vi "Echo Info.vi"(11 "Echo Info":string) -> (0 "Info Data":u16, 1 "Info Code":u16, 2 "FC":u8, 3 "Amplifier Num":u8, 4 "Check Result":bool)   [LabVIEW 2014, in "ALPHA5 RS485.lvlib"]
uses:
  ALPHA5 RS485.lvlib
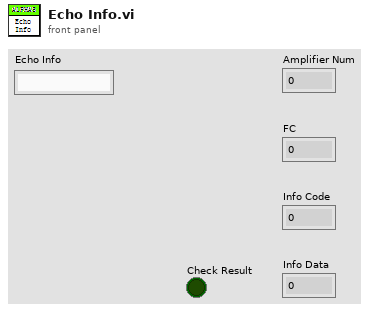
[diagram p1: front panel]
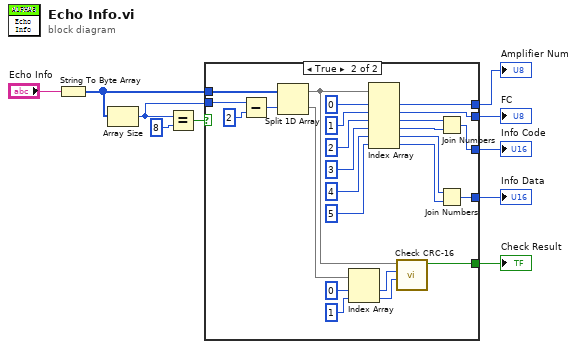
[diagram p0: block diagram]
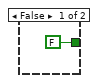
[diagram p2: hidden frame]
diagram:
  n1 = String To Byte Array(string="Echo Info") -> (unsigned byte array=w7:u8[])
  n2 = Array Size(array=w7) -> (size(s)=w6:i32)
  n3 = Equal?(x=w6, y=8) -> (x = y?=w8:bool)
  n4 = case shown="True" w8 {
    tunnel: w7 -> [_ w36]
    tunnel: w6 -> [_ w35]
    tunnel: [FALSE ("Check Result") w27] -> w5
    tunnel: [_ w21] -> w2
    tunnel: [_ w18] -> w1
    tunnel: [_ w13] -> w3
    tunnel: [_ w12] -> w4
    frame False {
    }
    frame True {
      n5 = Subtract(x=w35, y=2) -> (x-y=w33:i32)
      n6 = Split 1D Array(array=w36, index=w33) -> (first subarray=w22:u8[], second subarray=w32:u8[])
      n7 = Index Array(array=w32, index #1=0 ("index"), index #2=1 ("index")) -> (element #1=w29:u8, element #2=w28:u8)
      n8 = Index Array(array=w22, index #1=0 ("index"), index #2=1 ("index"), index #3=2 ("index"), index #4=3 ("index"), index #5=4 ("index"), index #6=5 ("index")) -> (element #1=w21:u8, element #2=w18:u8, element #3=w17:u8, element #4=w16:u8, element #5=w15:u8, element #6=w14:u8)
      n9 = call "Check CRC-16.vi"("CRC-16-H"=w28, "CRC-16-L"=w29, "Data In"=w22) -> ("Check Result"=w27:bool)  [unwired: 7 in, 1 out]
      n10 = Join Numbers(hi=w17, lo=w16) -> ((hi.lo)=w13:u16)
      n11 = Join Numbers(hi=w15, lo=w14) -> ((hi.lo)=w12:u16)
    }
  }
  "Check Result" <- w5
  "Amplifier Num" <- w2
  "Info Code" <- w3
  "Info Data" <- w4
  "FC" <- w1
